vi "Release Protected Subpanel.vi"(8 "error in (no error)":errorcluster, 11 "Protected Subpanel":T1) -> (0 "error out":errorcluster)   [LabVIEW 2017, in "IViewable.lvlib" / "ProtectedSubpanel.lvclass"]
uses:
  ProtectedSubpanel.lvclass
  Protected Subpanel Reference.ctl
  ProtectedSubpanel.lvclass/ProtectedSubpanel.ctl
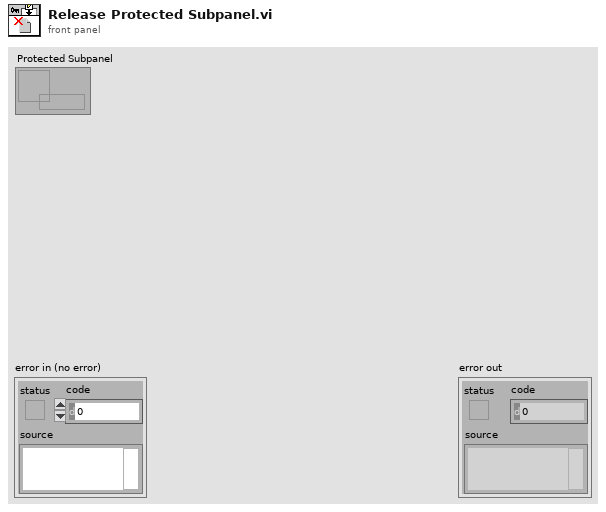
[diagram p1: front panel]
types:
  T1 = typedef "IViewable.lvlib/ProtectedSubpanel.lvclass/Protected Subpanel Reference.ctl" = refnum<data-value>
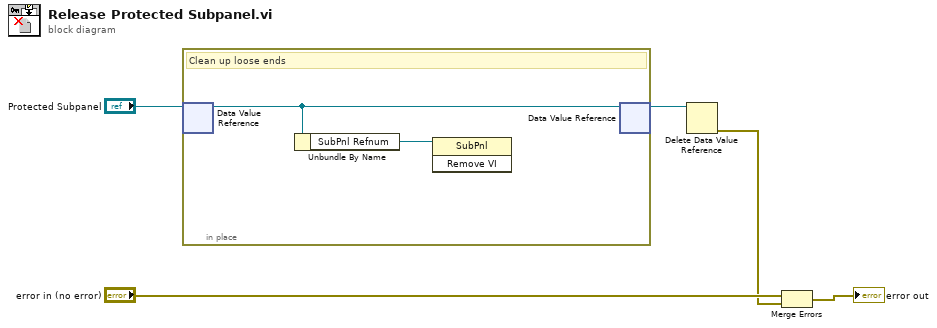
[diagram p0: block diagram]
diagram:
  n1 = in-place {
    # "Clean up loose ends"
    n2 = in-place-dvr #1("Protected Subpanel") -> (w7:refnum<class "ProtectedSubpanel.lvclass">)  [unwired: 1 out]
    n3 = Unbundle By Name(w7) -> ("SubPnl Refnum"=w6:refnum<vi>)
    n4 = invoke class="SubPnl" method="Remove VI"(reference=w6) -> ()  [unwired: 2 in, 3 out]
    n5 = in-place-dvr #1(w7) -> (w1:T1)  [unwired: 1 out]
  }
  n6 = Delete Data Value Reference(data value reference=w1) -> (error out=w3:errorcluster)  [unwired: 1 in, 1 out]
  n7 = Merge Errors("error in (no error)", w3) -> (→"error out":errorcluster)
